vi "GPS通讯(子VI).vi"(8 "error in (no error)":errorcluster caption="错误输入（无错误）") -> ()   [LabVIEW 2016, in "环境动力监测库.lvlib" / "NMEA.lvlib"]
uses:
  NMEA.lvlib
  <vilib>/Plasmionique/MB Master/MB_Master/MB_Master.lvclass
  <vilib>/Plasmionique/MB Master/MB_Master_TCP/MB_Master_TCP.lvclass
  C:/Program Files (x86)/National Instruments/LabVIEW 2016/vi.lib/Plasmionique/MB Master/MB_Master/MB_Master.lvclass
  <vilib>/Instr/_visa.llb/VISA Configure Serial Port (Instr).vi
  <vilib>/Plasmionique/MB Master/MB Master.lvlib
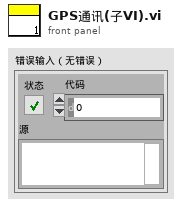
[diagram p1: front panel]
types:
  T1 = cluster{"定位状态":bool, "卫星数量":u16, "时间标识":timestamp, "纬度":dbl, "南北":string, "经度":dbl, "东西":string}
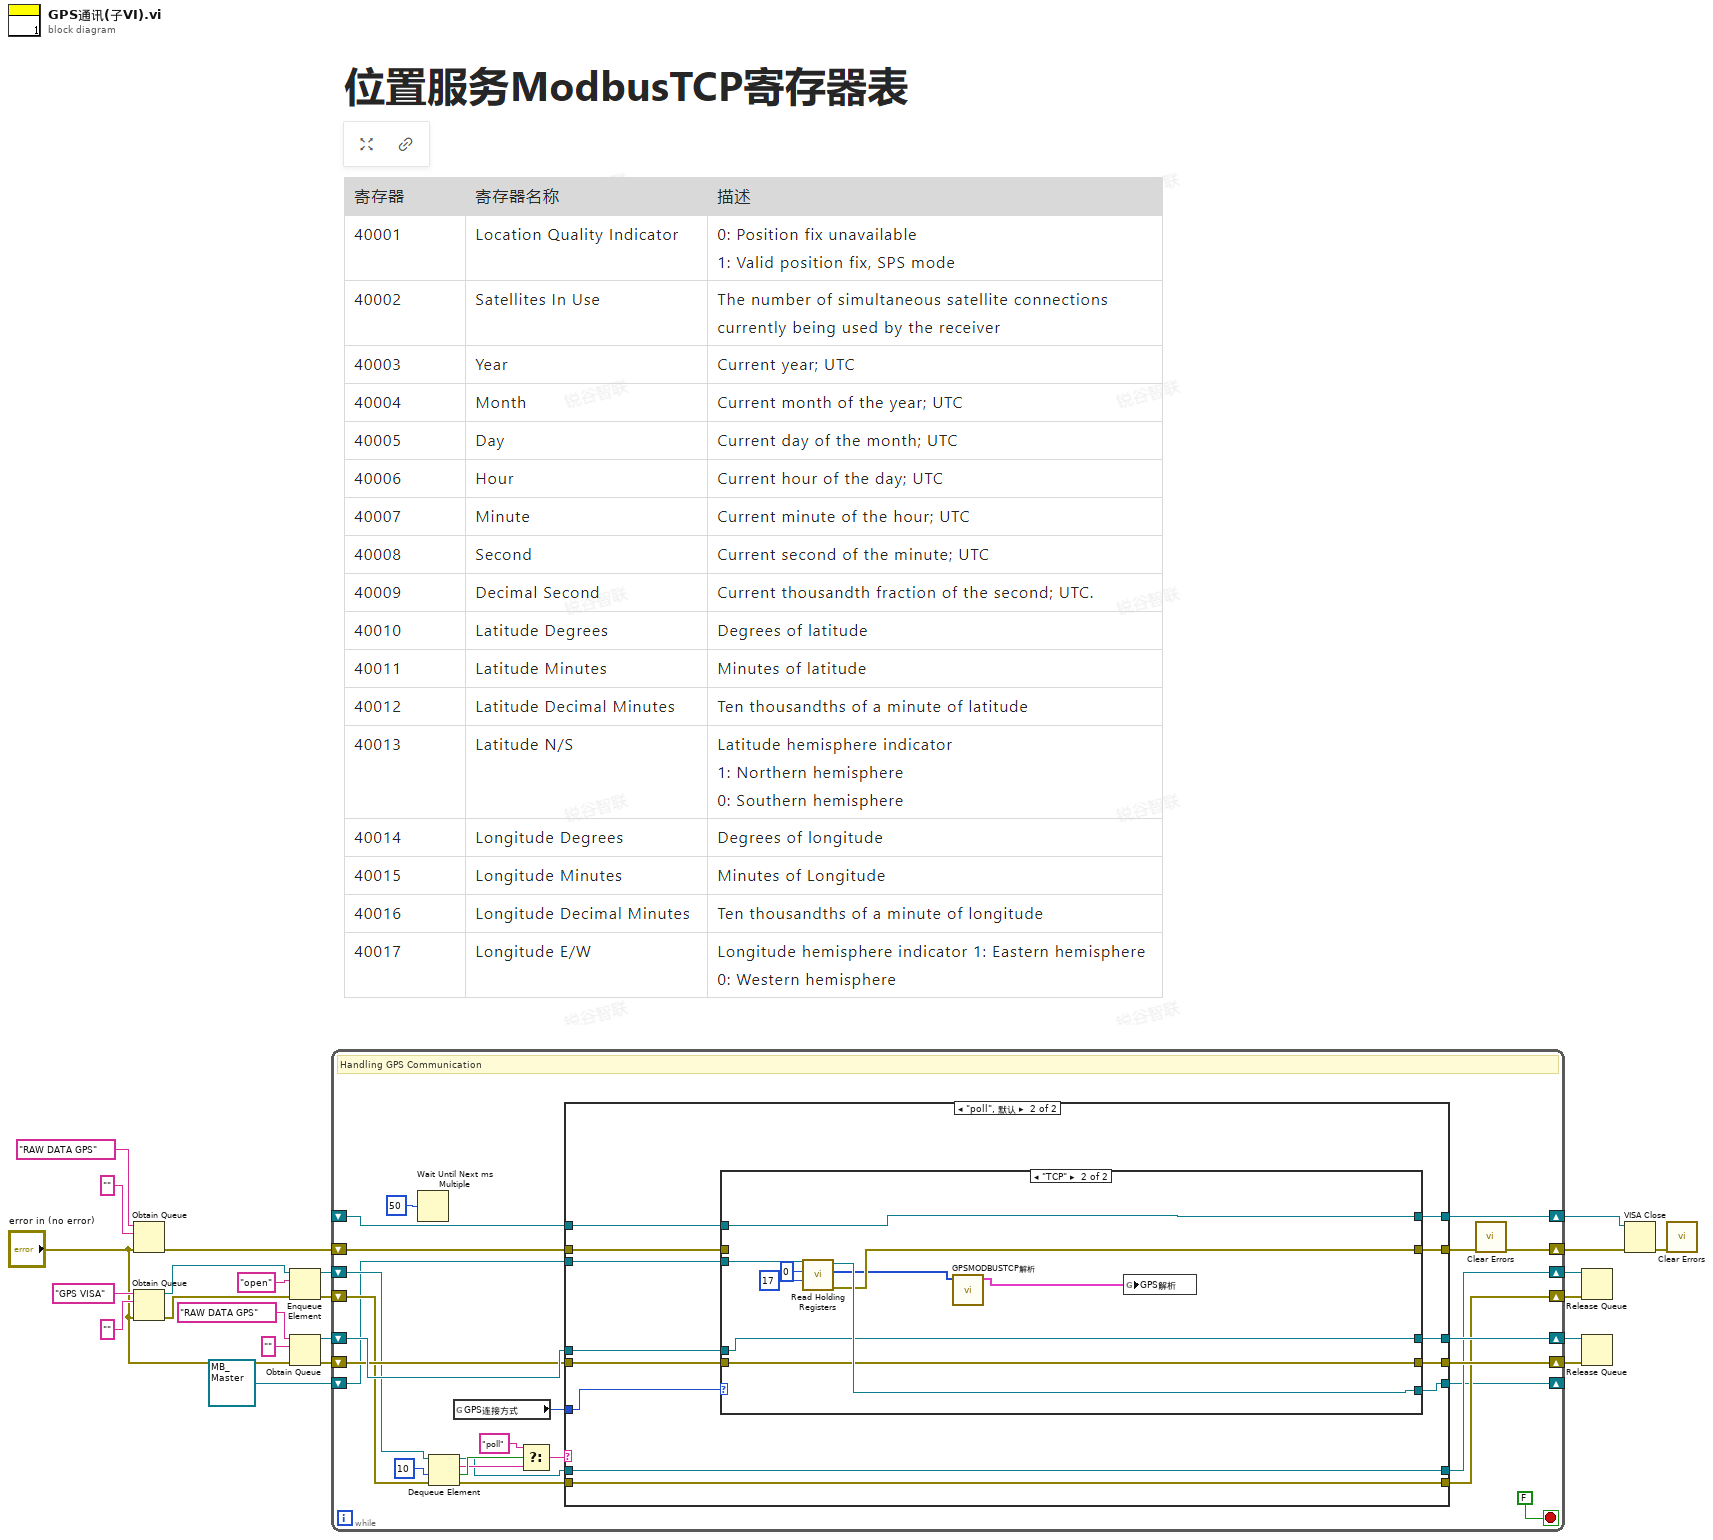
[diagram p0: block diagram]
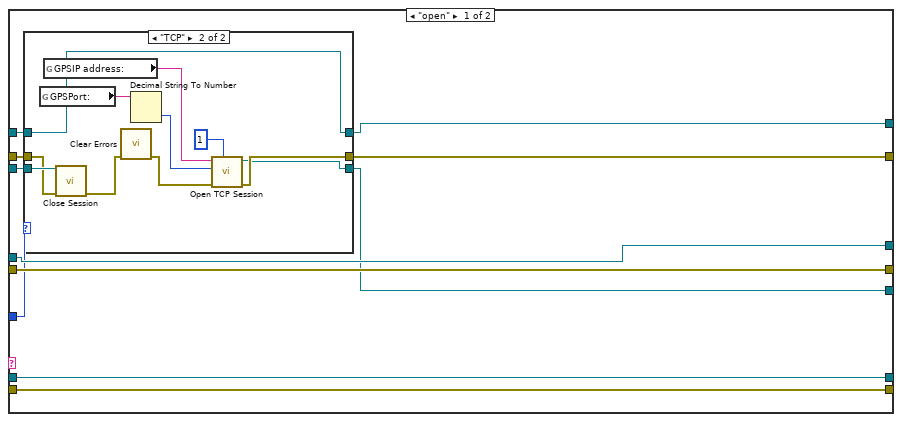
[diagram p2: hidden frame]
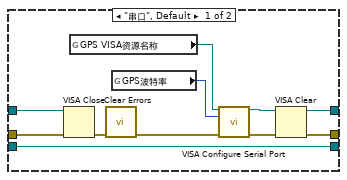
[diagram p3: hidden frame]
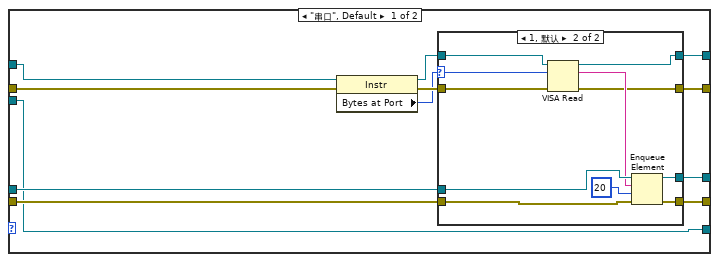
[diagram p4: hidden frame]
diagram:
  n1 = Obtain Queue(name (unnamed)="RAW DATA GPS" ("nom (aucun)"), element data type="" ("expression régulière"), error in (no error)="error in (no error)") -> (error out=w14:errorcluster)  [unwired: 2 in, 2 out]
  n2 = Obtain Queue(name (unnamed)="GPS VISA" ("名称（未命名）"), element data type="" ("名称（未命名）"), error in (no error)="error in (no error)") -> (queue out=w11:refnum<queue>, error out=w10:errorcluster)  [unwired: 2 in, 1 out]
  n3 = Enqueue Element(queue=w11, element="open" ("元素"), error in (no error)=w10) -> (queue out=w8:refnum<queue>, error out=w7:errorcluster)  [unwired: 1 in, 1 out]
  n4 = Obtain Queue(name (unnamed)="RAW DATA GPS" ("nom (aucun)"), element data type="" ("expression régulière"), error in (no error)="error in (no error)") -> (queue out=w4:refnum<queue>, error out=w3:errorcluster)  [unwired: 2 in, 1 out]
  n5 = while {
    shift-right: [w45] -> w18
    shift-left: w3 -> [w47]
    shift-right: [w44] -> w20
    shift-left: _ -> [w43]
    shift-right: [w46] -> w19
    shift-left: w4 -> [w48]
    shift-right: [w39] -> w21
    shift-left: w14 -> [w41]
    shift-right: [w29] -> w22
    shift-left: w7 -> [w37]
    shift-right: [w31] -> w23
    shift-left: w8 -> [w38]
    shift-right: [w25] -> _
    shift-left: refnum<class "MB_Master.lvclass"> refnum ("MB session in") -> [w24]
    stop <- FALSE stop-if-true
    # "Handling GPS Communication"
    n6 = Wait Until Next ms Multiple(millisecond multiple=u32 50 ("attente (ms)")) -> ()  [unwired: 1 out]
    n7 = Dequeue Element(queue=w38, timeout in ms (-1)=10 ("超时毫秒(-1)"), error in (no error)=w37) -> (queue out=w30:refnum<queue>, element=w33:string, timed out?=w35:bool, error out=w28:errorcluster)
    n8 = global read "断电保存全局变量.vi" "GPS连接方式"() -> (w26:enum16{"串口", "TCP"})
    n9 = Select(t="poll" ("名称（未命名）"), s=w35, f=w33) -> (s? t:f=w32:string)
    n10 = case shown="\"poll\", 默认" w32 {
      tunnel: w48 -> [w57 w94]
      tunnel: w47 -> [w56 w93]
      tunnel: [w57 w92] -> w46
      tunnel: [w56 w91] -> w45
      tunnel: [w53 w90] -> w44
      tunnel: w43 -> [w54 w89]
      tunnel: w41 -> [w55 w88]
      tunnel: [w52 w87] -> w40
      tunnel: [w59 w86] -> w31
      tunnel: w30 -> [w59 w86]
      tunnel: [w58 w85] -> w29
      tunnel: w28 -> [w58 w85]
      tunnel: w26 -> [w51 w84]
      tunnel: [w50 w82] -> w25
      tunnel: w24 -> [w49 w83]
      frame "open" {
        n11 = case shown="\"TCP\"" w51 {
          tunnel: w55 -> [w67 w73]
          tunnel: w54 -> [w66 w81]
          tunnel: [w63 w81] -> w53
          tunnel: [w61 w75] -> w52
          tunnel: [w60 w71] -> w50
          tunnel: w49 -> [w60 w74]
          frame "串口", Default {
            n12 = VISA Close(VISA resource name=w66, error in (no error)=w67) -> (error out=w65:errorcluster)
            n13 = global read "断电保存全局变量.vi" "GPS VISA资源名称"() -> (w69:refnum<visa-resource-name>)
            n14 = call <vilib>:"Clear Errors.vi"("error in (no error)"=w65) -> ("error out"=w64:errorcluster)  [unwired: 5 in, 1 out]
            n15 = global read "断电保存全局变量.vi" "GPS波特率"() -> (w70:u32)
            n16 = call-poly "VISA Configure Serial Port"("VISA resource name"=w69, "baud rate (9600)"=w70, "error in (no error)"=w64) -> ("VISA resource name out"=w68:refnum<visa-resource-name>, "error out"=w62:errorcluster)  [unwired: 11 in]
            n17 = VISA Clear(VISA resource name=w68, error in (no error)=w62) -> (VISA resource name out=w63:refnum<visa-resource-name>, error out=w61:errorcluster)
          }
          frame "TCP" {
            n18 = global read "断电保存全局变量.vi" "GPSPort:"() -> (w78:string)
            n19 = global read "断电保存全局变量.vi" "GPSIP address:"() -> (w79:string)
            n20 = call-dynamic "Close Session.vi"("error in (no error)"=w73, "MB session in"=w74) -> ("error out"=w72:errorcluster)  [unwired: 9 in]
            n21 = call <vilib>:"Clear Errors.vi"("error in (no error)"=w72) -> ("error out"=w76:errorcluster)  [unwired: 5 in, 1 out]
            n22 = Decimal String To Number(string=w78) -> (number=w77:i32)  [unwired: 2 in, 1 out]
            n23 = call <vilib>:"Open TCP Session.vi"("Slave ID (255)"=u8 1, "error in (no error)"=w76, "Port (502)"=w77, "IP Address"=w79) -> ("error out"=w75:errorcluster, "MB_TCP session"=w71:refnum<class "MB_Master_TCP.lvclass">)  [unwired: 6 in]
          }
        }
      }
      frame "poll", Default {
        n24 = case shown="\"TCP\"" w84 {
          tunnel: w94 -> [w106 w125]
          tunnel: w93 -> [w105 w124]
          tunnel: [w104 w125] -> w92
          tunnel: [w103 w124] -> w91
          tunnel: [w102 w131] -> w90
          tunnel: w89 -> [w101 w131]
          tunnel: w88 -> [w100 _]
          tunnel: [w99 w126] -> w87
          tunnel: w83 -> [w95 w130]
          tunnel: [w95 w127] -> w82
          frame "串口", Default {
            n25 = property class="Instr"(reference=w101, error in=w100) -> (reference out=w98:refnum<visa-resource-name>, error out=w97:errorcluster, "Bytes at Port"=w96:u32)
            n26 = case shown="1, 默认" w96 {
              selector: w96 -> [_ w112]
              tunnel: w106 -> [w107 w121]
              tunnel: w105 -> [w108 w120]
              tunnel: [w107 w119] -> w104
              tunnel: [w108 w118] -> w103
              tunnel: [w109 w116] -> w102
              tunnel: w98 -> [w109 w115]
              tunnel: w97 -> [w110 w114]
              tunnel: [w110 w113] -> w99
              frame 0 {
              }
              frame 1, Default {
                n27 = VISA Read(VISA resource name=w115, byte count=w112, error in (no error)=w114) -> (VISA resource name out=w116:refnum<visa-resource-name>, read buffer=w117:string, error out=w113:errorcluster)  [unwired: 1 out]
                n28 = Enqueue Element(queue=w121, element=w117, timeout in ms (-1)=20 ("timeout en ms (-1)"), error in (no error)=w120) -> (queue out=w119:refnum<queue>, error out=w118:errorcluster)  [unwired: 1 out]
              }
            }
          }
          frame "TCP" {
            n29 = call <vilib>:"Read Holding Registers.vi"("quantity"=u16 17, "starting address"=u16 0, "MB session in"=w130) -> ("error out"=w126:errorcluster, "Registers"=w123:u16[], "MB session out"=w127:refnum<class "MB_Master.lvclass">)  [unwired: 6 in]
            n30 = call "GPSMODBUSTCP解析.vi"("Registers"=w123) -> ("GPS解析"=w122:T1)  [unwired: 10 in]
            n31 = global write "NMEA过程全局变量.vi" "GPS解析"(w122) -> ()
          }
        }
      }
    }
    n32 = call <vilib>:"Clear Errors.vi"("error in (no error)"=w40) -> ("error out"=w39:errorcluster)  [unwired: 5 in, 1 out]
  }
  n33 = Release Queue(queue=w23, error in (no error)=w22) -> ()  [unwired: 1 in, 3 out]
  n34 = Release Queue(queue=w19, error in (no error)=w18) -> ()  [unwired: 1 in, 3 out]
  n35 = VISA Close(VISA resource name=w20, error in (no error)=w21) -> (error out=w17:errorcluster)
  n36 = call <vilib>:"Clear Errors.vi"("error in (no error)"=w17) -> ()  [unwired: 5 in, 2 out]
